vi "squiggle_calibrate.vi"(8 "error in":errorcluster, 11 "I2C interface":T1) -> (0 "error out":errorcluster)   [LabVIEW 2013]
uses:
  i2c_interface.ctl
  fpga_reference.ctl
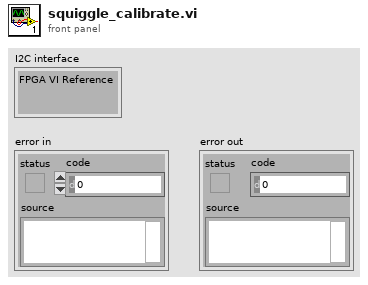
[diagram p1: front panel]
types:
  T1 = typedef "i2c_interface.ctl" = cluster{"FPGA VI Reference":T2}
  T2 = typedef "fpga_reference.ctl" = refnum<k20>
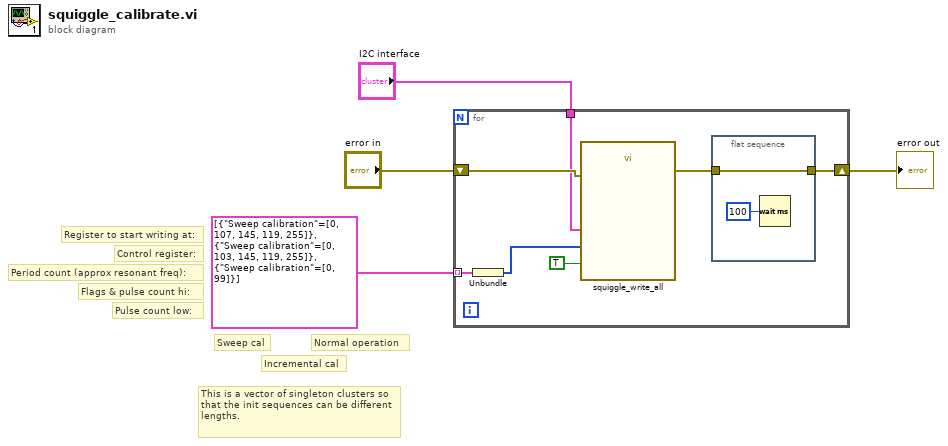
[diagram p0: block diagram]
diagram:
  # "Period count (approx resonant freq):"
  # "Pulse count low:"
  # "Flags & pulse count hi:"
  # "Control register:"
  # "Register to start writing at:"
  # "This is a vector of singleton clusters so that the init sequences can be different lengths."
  # "Normal operation"
  # "Incremental cal"
  # "Sweep cal"
  n1 = for {
    tunnel: "I2C interface" -> [w8]
    tunnel: cluster{"Sweep calibration":u8[]}[] [{"Sweep calibration"=[0, 107, 145, 119, 255]}, {"Sweep calibration"=[0, 103, 145, 119, 255]}, {"Sweep calibration"=[0, 99]}] -> [w7] mode=indexing
    shift-right: [w5] -> w3
    shift-left: "error in" -> [w11]
    n2 = Unbundle(w7) -> ("Sweep calibration"=w6:u8[])
    n3 = call "squiggle_write_all.vi"("Init sequence"=w6, "Error in"=w11, "Send init sequence"=TRUE, "I2C interface"=w8) -> ("Error out"=w9:errorcluster)  [unwired: 7 in]
    n4 = flat-sequence {
      tunnel: w9 -> [w13]
      tunnel: [w13] -> w5
      frame #0 {
        n5 = Wait (ms)(milliseconds to wait=u32 100) -> ()  [unwired: 1 out]
      }
    }
  }
  "error out" <- w3
